vi "上管柱上转向轴合成.vi"() -> ()   [LabVIEW 2018]
uses:
  Global_Variable/Global.vi
  Database/Global1.vi
  Global_Variable/A131258.vi
  <vilib>/addons/database/Connection.llb/DB Tools Open Connec (String).vi
  <vilib>/addons/database/Connection.llb/Conn Execute.vi
  <vilib>/addons/database/Recordset.llb/Rec Fetch Recordset Data (R).vi
  <vilib>/Utility/config.llb/NI_LVConfig.lvlib
  <vilib>/addons/database/NI_Database_API.lvlib
panel:
  out "Fdeviceid":string
  out "USER_ID":string
  out "deviceid":string
  out "productid":string
  out "产品型号":string
  out "codeid":string
  out "联机模式":string
  out "用户权限":string
  out "用户名":string
  in  "上转向轴拉装报表":string[][](table)=[["mm"], ["mm/s"]]
  in  "上转向轴拉装判定结果":bool[][](array[boolean])=[[TRUE]]
  in  "选项卡控件 2":enum32{"上转向轴拉装曲线", "参数查看"}(tab)
  out "上序状态显示":string
  out "上序状态":bool
  in  "质量报警":bool
  in  "设备缺料":bool
  in  "设备故障":bool
  out "CCD卡簧检测":string
  out "判定结果3":string
  out "判定结果2":string
  out "判定结果1":string
  out "最终位移上限":dbl
  out "最终位移下限":dbl
  out "最小压力上限":dbl
  out "最小压力下限":dbl
  out "最大压力上限":dbl
  out "最大压力下限":dbl
  out "拉装最终位移(mm)":dbl
  out "不合格指示灯":bool
  out "合格指示灯":bool
  out "拉力位移曲线":cluster{dbl[], dbl[]}[](graph)
  out "位移区间内最大压力(KN)":dbl
  out "位移区间内最小压力(KN)":dbl
  out "产品条码":string
  in  "删除":bool
  in  "确定":bool
  in  "添加":bool
  in  "退出":bool
  in  "更新":bool
  in  "产品型号":string(combo)
  in  "选项卡控件 3":enum32{"上转向轴拉装参数", "产品管理", "用户管理"}(tab)
  in  "坐标轴参数":string[][](table)=[["mm"], ["mm/s"]]
  in  "判定框参数":string[][](table)=[["mm"], ["mm/s"]]
  in  "结果判定参数":string[][](table)=[["mm"], ["mm/s"]]
  in  "请输入添加的产品名称":string
  in  "请选择要删除的产品":string(combo)
  in  "进入用户管理":bool
  # "160上管柱上转向轴合成"
  # "下限值"
  # "上限值"
  # "拉装结果"
  # "判定结果"
  # "生产结果"
  # "产品二维码"
  # "上序状态："
  # "CCD卡簧检测结果"
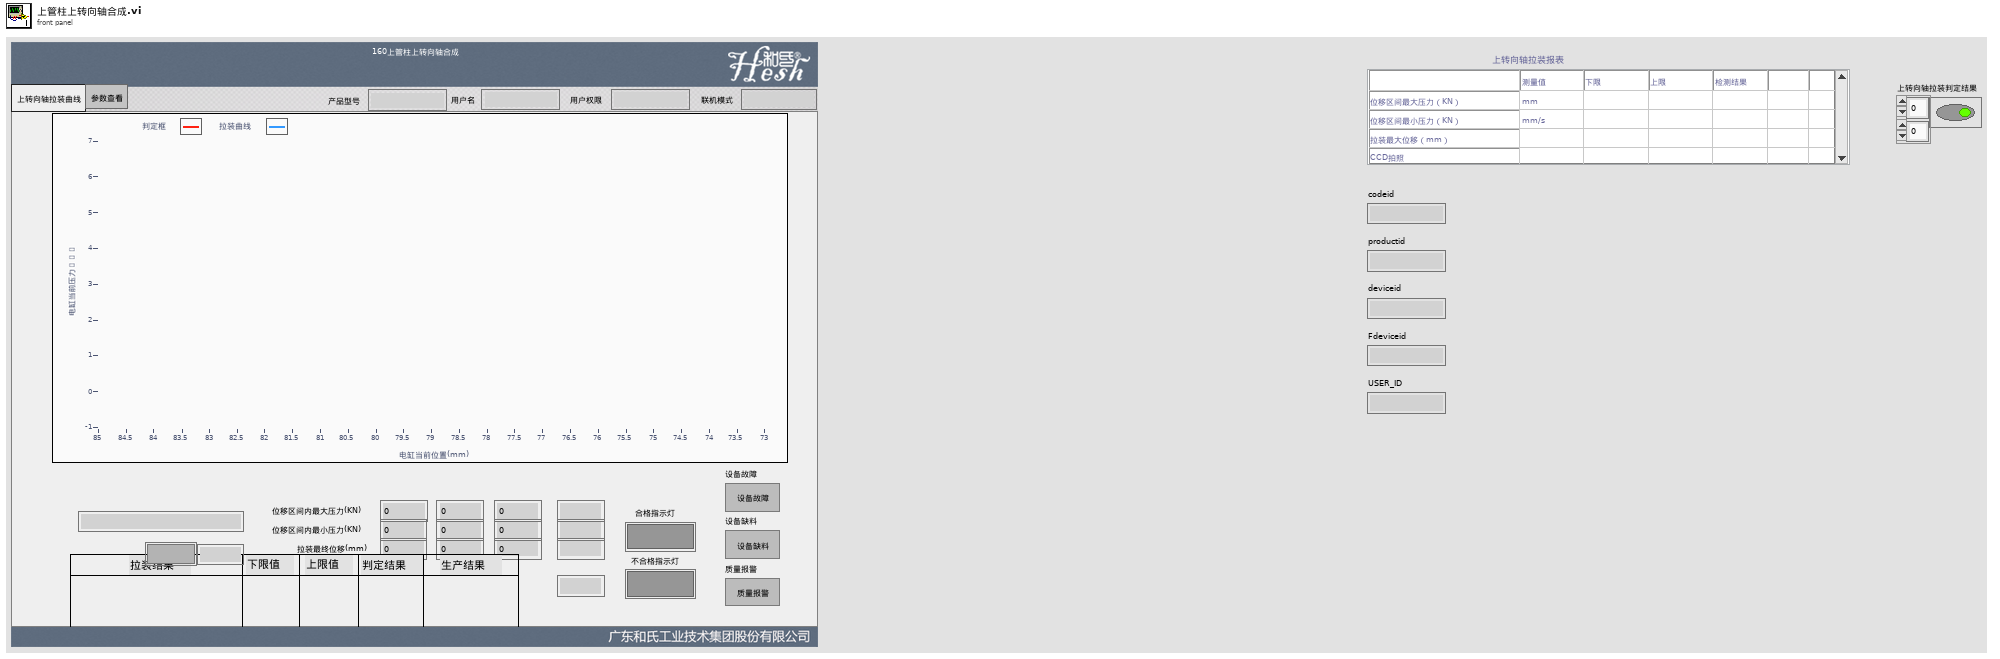
[diagram p1: front panel]
types:
  T1 = enum32{"Invalid", "Standard", "Closed", "Hidden", "Minimized", "Maximized"}
  T2 = cluster{"用户编号":string, "用户名":string, "用户密码(密文)":string, "用户权限":string}
  T3 = cluster{"设备名称":string, "用户名":string, "设备状态":enum16{"设备离线", "设备正常", "设备缺料", "设备故障", "质量报警"}, "附加信息":string}
  T4 = typedef "NI_LVConfig.lvlib/Config Data RefNum.ctl" = refnum<k1>
  T5 = cluster{i64, i64, string, "位移区间内最小压力(KN)":dbl, "最小压力下限":dbl, "最小压力上限":dbl, string, "判定结果2":string}
  T6 = cluster{i64, i64, string, "拉装最终位移(mm)":dbl, "最终位移下限":dbl, "最终位移上限":dbl, string, "判定结果3":string}
  T7 = cluster{i64, i64, string, dbl, dbl, dbl, string, "元素":string}
  T8 = cluster{i64, i64, string, "位移区间内最大压力(KN)":dbl, "最大压力下限":dbl, "最大压力上限":dbl, string, "判定结果1":string}
  T9 = cluster{i64, i64, string, "拉装最终位移(mm)":dbl, "最终位移下限":dbl, "最终位移上限":dbl, string, "元素":string}[]
  T10 = typedef "NI_Database_API.lvlib/Conn ObjectReference.ctl" = refnum<k1>
  T11 = cluster{i64, i64, "拉装最终位移(mm)":dbl, "最终位移下限":dbl, "最终位移上限":dbl, string, "元素":string}
  T12 = cluster{i64, i64, i64, string, "result string":string}
  T13 = cluster{i64, i64, i64, string, "result string":string}[]
  T14 = typedef "NI_Database_API.lvlib/Rec ObjectReference.ctl" = refnum<k1>
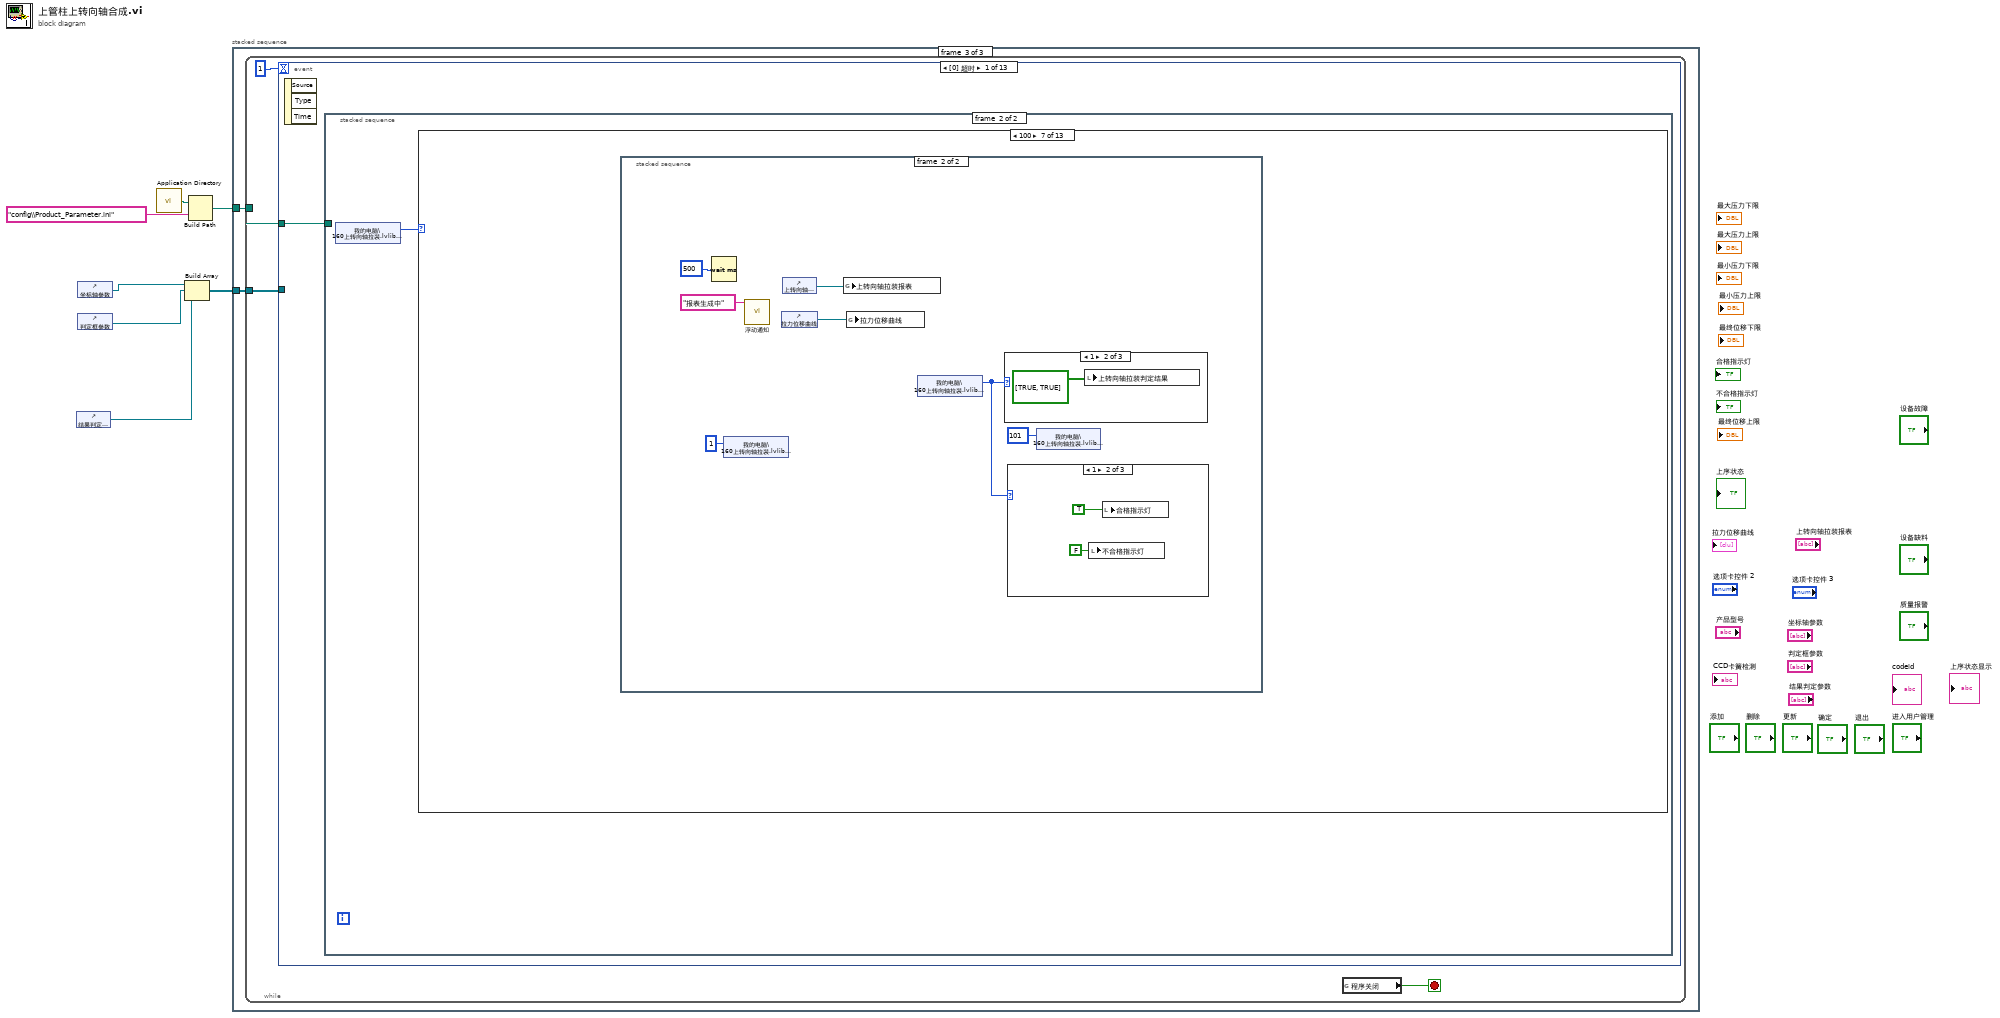
[diagram p0: block diagram]
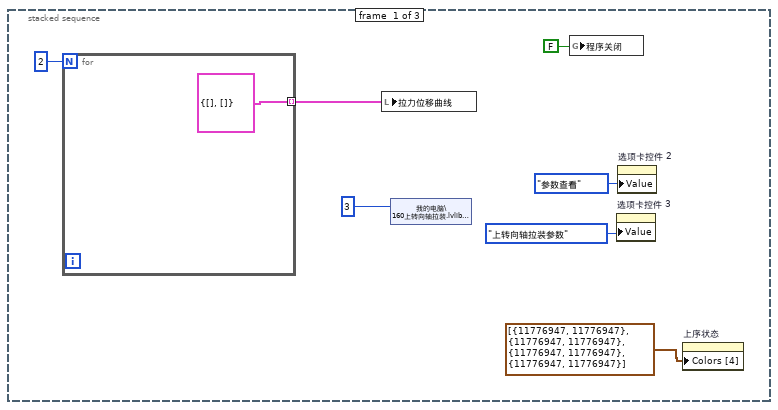
[diagram p2: hidden frame]
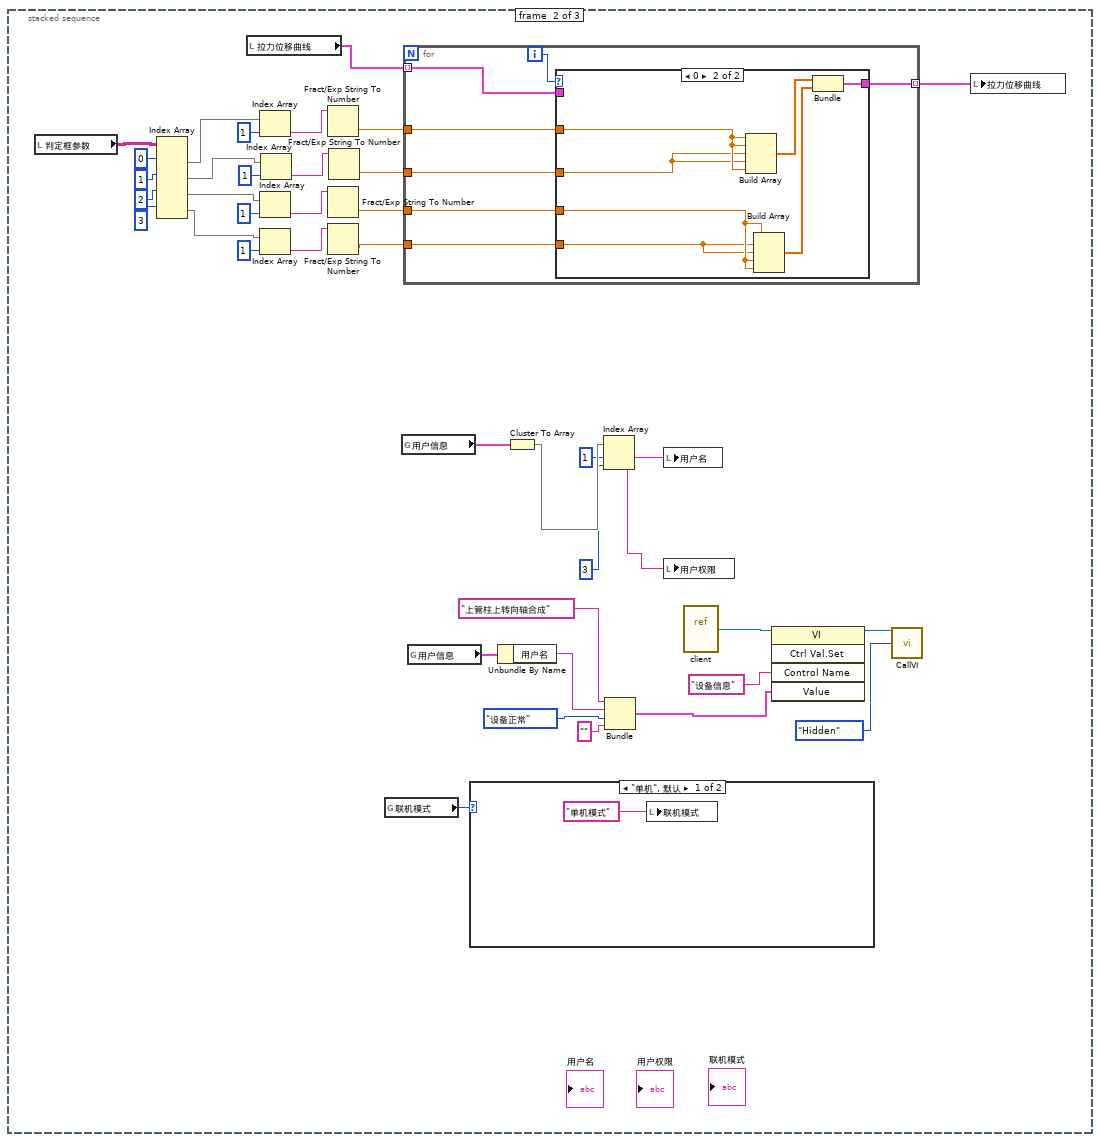
[diagram p3: hidden frame]
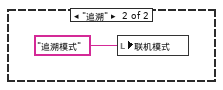
[diagram p4: hidden frame]
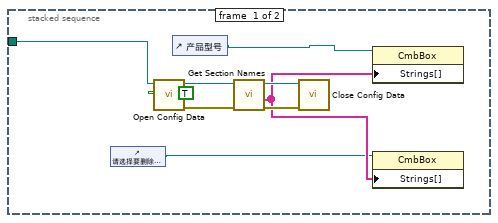
[diagram p6: hidden frame]
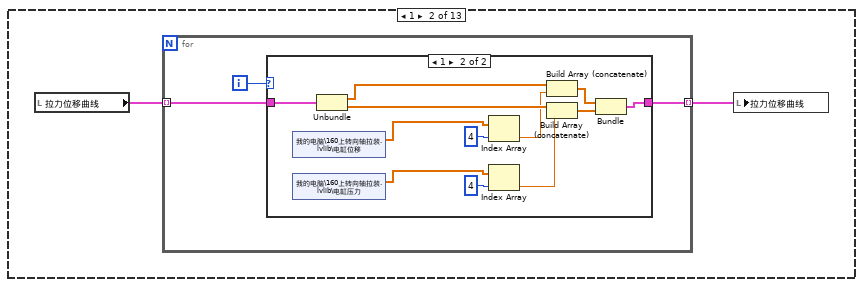
[diagram p8: hidden frame]
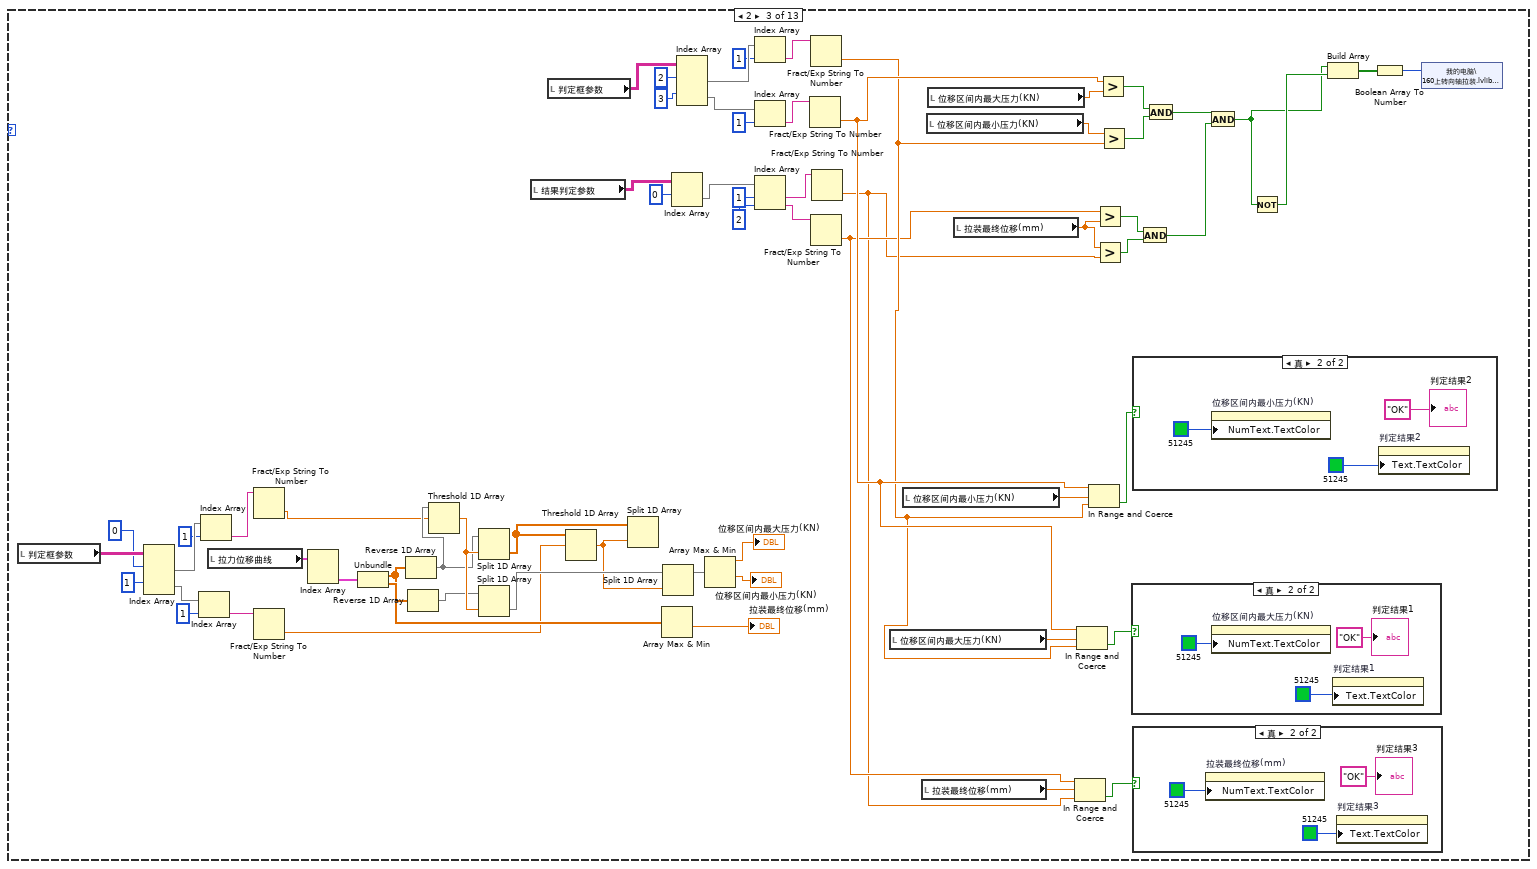
[diagram p10: hidden frame]
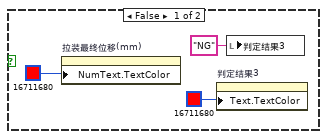
[diagram p11: hidden frame]
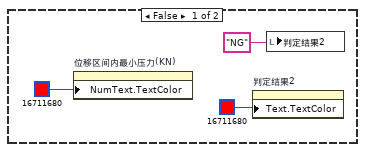
[diagram p12: hidden frame]
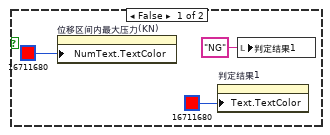
[diagram p13: hidden frame]
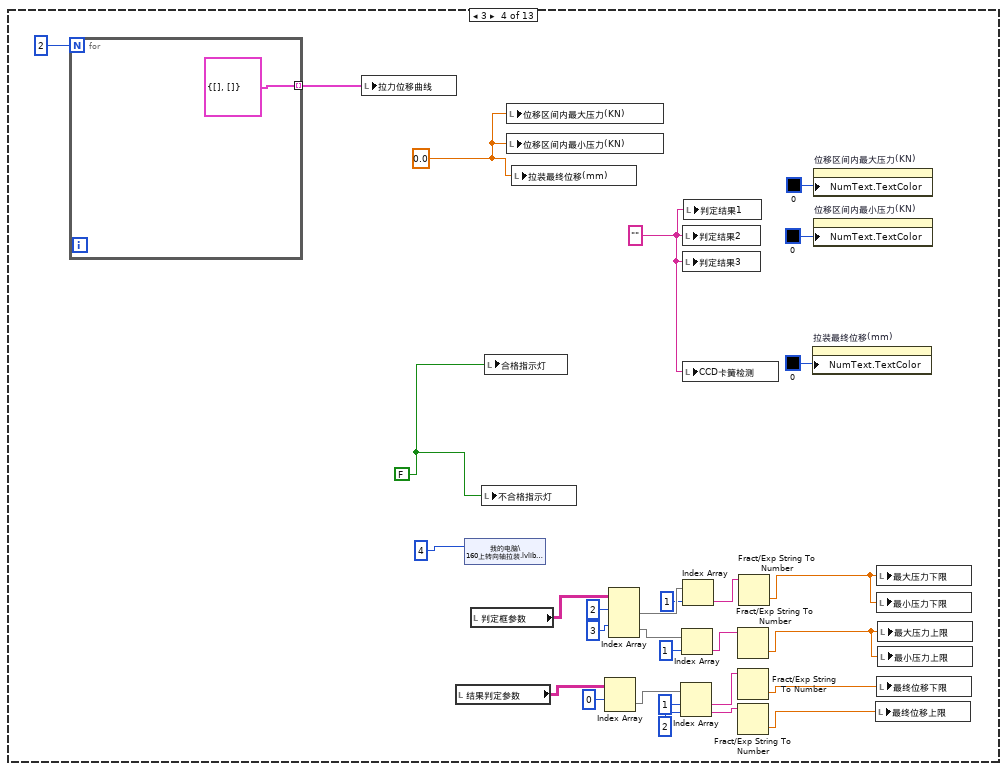
[diagram p14: hidden frame]
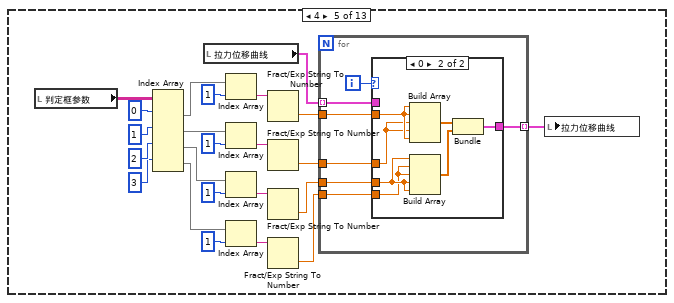
[diagram p15: hidden frame]
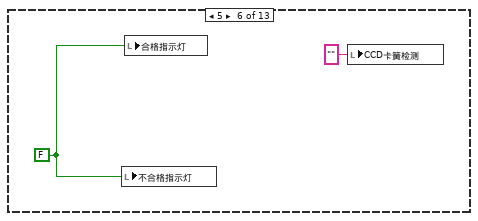
[diagram p17: hidden frame]
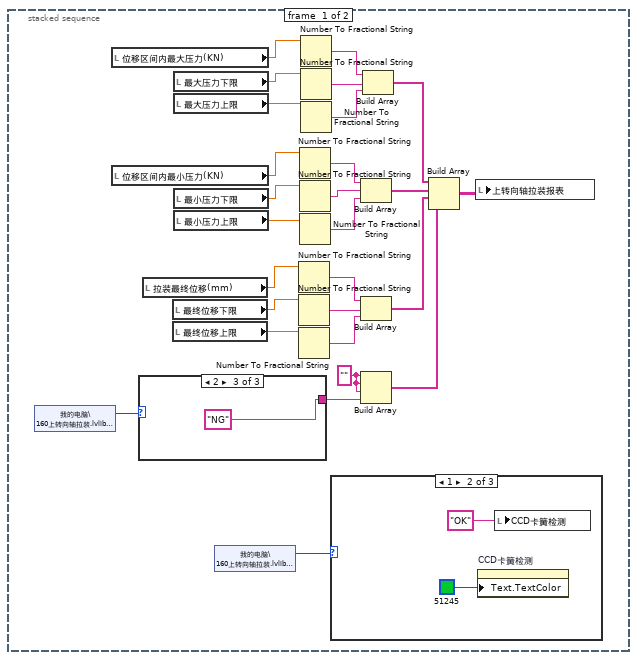
[diagram p18: hidden frame]
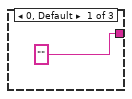
[diagram p19: hidden frame]
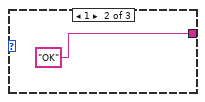
[diagram p20: hidden frame]
diagram:
  n1 = control-ref of="结果判定参数"() -> (w2:refnum<vi>)
  n2 = control-ref of="坐标轴参数"() -> (w4:refnum<vi>)
  n3 = control-ref of="判定框参数"() -> (w3:refnum<vi>)
  n4 = call <vilib>:"Application Directory.vi"() -> ("Application Directory"=w7:path)
  n5 = Build Array(w4, w3, w2) -> (w1:refnum<vi>[])
  n6 = Build Path(base path=w7, name or relative path="config\\Product_Parameter.ini" ("名称或相对路径")) -> (appended path=w5:path)
  n7 = stacked-sequence {
    tunnel: w5 -> [_ _ w74]
    tunnel: w1 -> [_ _ w73]
    frame #0 {
      n8 = for {
        N: 2 -> [_]
        tunnel: [cluster{dbl[], dbl[]} {[], []}] -> w14 mode=indexing
      }
      n9 = local write "拉力位移曲线"(w14) -> ()
      n10 = shared-variable "我的电脑\\160上转向轴拉装.lvlib\\备用_1"(3) -> ()  [unwired: 1 in, 1 out]
      n11 = global write "Global.vi" "程序关闭"(FALSE ("程序关闭")) -> ()
      n12 = property on="选项卡控件 3" class="TabCtl (严格)"("Value"=enum32{"上转向轴拉装参数", "产品管理", "用户管理"}."上转向轴拉装参数" ("选项卡控件 3")) -> ()  [unwired: 2 in, 2 out]
      n13 = property on="选项卡控件 2" class="TabCtl (严格)"("Value"=enum32{"上转向轴拉装曲线", "参数查看"}."参数查看" ("选项卡控件 2")) -> ()  [unwired: 2 in, 2 out]
      n14 = property on="上序状态" class="Bool (严格)"("Colors [4]"=cluster{u32, u32}[] [{11776947, 11776947}, {11776947, 11776947}, {11776947, 11776947}, {11776947, 11776947}] ("颜色[4]")) -> ()  [unwired: 2 in, 2 out]
    }
    frame #1 {
      n15 = local read "判定框参数"() -> (w53:string[][])
      n16 = Index Array(array=w53, index (row) #1=0 ("索引 (行)"), index (row) #2=1 ("索引 (行)"), index (row) #3=2 ("索引 (行)"), index (row) #4=3 ("索引 (行)")) -> (element #1=w48:string[], element #2=w43:string[], element #3=w38:string[], element #4=w34:string[])  [unwired: 4 in]
      n17 = local read "拉力位移曲线"() -> (w55:cluster{dbl[], dbl[]}[])
      n18 = Index Array(array=w48, index=1 ("索引")) -> (element=w46:string)
      n19 = Index Array(array=w38, index=1 ("索引")) -> (element=w39:string)
      n20 = Index Array(array=w34, index=1 ("索引")) -> (element=w35:string)
      n21 = Index Array(array=w43, index=1 ("索引")) -> (element=w42:string)
      n22 = Fract/Exp String To Number(string=w46) -> (number=w45:dbl)  [unwired: 3 in, 1 out]
      n23 = Fract/Exp String To Number(string=w39) -> (number=w37:dbl)  [unwired: 3 in, 1 out]
      n24 = Fract/Exp String To Number(string=w35) -> (number=w33:dbl)  [unwired: 3 in, 1 out]
      n25 = Fract/Exp String To Number(string=w42) -> (number=w41:dbl)  [unwired: 3 in, 1 out]
      n26 = global read "Global1.vi" "联机模式"() -> (w27:enum16{"单机", "追溯"})
      n27 = global read "Global1.vi" "用户信息"() -> (w23:T2)
      n28 = for {
        tunnel: [w64] -> w54 mode=indexing
        tunnel: w55 -> [w63] mode=indexing
        tunnel: w45 -> [w61]
        tunnel: w41 -> [w60]
        tunnel: w37 -> [w59]
        tunnel: w33 -> [w58]
        i -> [w62]
        n29 = case shown="0" w62 {
          tunnel: [w65 w70] -> w64
          tunnel: w63 -> [w65 _]
          tunnel: w61 -> [_ w69]
          tunnel: w60 -> [_ w68]
          tunnel: w59 -> [_ w67]
          tunnel: w58 -> [_ w66]
          frame Default {
          }
          frame 0 {
            n30 = Build Array(w69, w69, w68, w68, w69) -> (w71:dbl[])
            n31 = Build Array(w67, w66, w66, w67, w67) -> (w72:dbl[])
            n32 = Bundle(w71, w72) -> (w70:cluster{dbl[], dbl[]})  [unwired: 1 in]
          }
        }
      }
      n33 = global read "Global1.vi" "用户信息"() -> (w30:T2)
      n34 = case shown="\"单机\", 默认" w27 {
        frame "单机", Default {
          n35 = local write "联机模式"("单机模式" ("联机模式")) -> ()
        }
        frame "追溯" {
          n36 = local write "联机模式"("追溯模式" ("联机模式")) -> ()
        }
      }
      n37 = Unbundle By Name(w30) -> ("用户名"=w31:string)
      n38 = Cluster To Array(cluster=w23) -> (array=w24:string[])
      n39 = Index Array(array=w24, index #1=1 ("索引"), index #2=3 ("索引")) -> (element #1=w25:string, element #2=w26:string)
      n40 = Bundle("设备名称"="上管柱上转向轴合成", "用户名"=w31, "设备状态"=enum16{"设备离线", "设备正常", "设备缺料", "设备故障", "质量报警"}."设备正常", "附加信息"="") -> (w32:T3)  [unwired: 1 in]
      n41 = local write "用户名"(w25) -> ()
      n42 = local write "用户权限"(w26) -> ()
      n43 = vi-ref "client.vi"() -> (w28:refnum<vi>)
      n44 = invoke class="VI" method="Ctrl Val.Set"(reference=w28, "Control Name"="设备信息" ("控件名"), "Value"=w32) -> (reference out=w29:refnum<vi>)  [unwired: 2 in, 4 out]
      n45 = call "CallVI.vi"("VI引用"=w29, "状态"=T1."Hidden") -> ()  [unwired: 11 in, 3 out]
      n46 = local write "拉力位移曲线"(w54) -> ()
    }
    frame #2 {
      n47 = while {
        tunnel: w74 -> [w77]
        tunnel: w73 -> [w78]
        stop <- w75 stop-if-true
        n48 = event shown="[0] 超时" {
          selector: _ -> [_ _ _ _ _ _ _ _ _ _ _ _ _]
          dyn-events: _ -> [_ _ _ _ _ _ _ _ _ _ _ _ _]
          timeout: 1 -> [_ _ _ _ _ _ _ _ _ _ _ _ _]
          tunnel: w77 -> [w79 w546 _ w679 w696 _ w707 _ _ _ _ _ _]
          tunnel: w78 -> [_ _ _ w677 w695 _ w706 _ _ _ _ _ _]
          event Timeout {
            n49 = event-data() -> ()  [unwired: 1 in, 3 out]
            n50 = stacked-sequence {
              tunnel: w79 -> [w82 _]
              frame #0 {
                n51 = control-ref of="请选择要删除的产品"() -> (w81:refnum<vi>)
                n52 = call <vilib>:"Open Config Data.vi"("create file if necessary (T)"=TRUE, "configuration file path"=w82) -> ("error out"=w85:errorcluster, "refnum"=w84:T4)  [unwired: 7 in, 1 out]
                n53 = control-ref of="产品型号"() -> (w80:refnum<vi>)
                n54 = call <vilib>:"Get Section Names.vi"("error in (no error)"=w85, "refnum"=w84) -> ("error out"=w87:errorcluster, "section names"=w83:string[], "refnum out"=w86:T4)  [unwired: 7 in]
                n55 = call <vilib>:"Close Config Data.vi"("error in (no error)"=w87, "refnum"=w86) -> ()  [unwired: 8 in, 2 out]
                n56 = property on="属性节点" class="CmbBox"(reference=w80, "Strings[]"=w83) -> ()  [unwired: 1 in, 2 out]
                n57 = property on="属性节点" class="CmbBox"(reference=w81, "Strings[]"=w83) -> ()  [unwired: 1 in, 2 out]
              }
              frame #1 {
                n58 = shared-variable "我的电脑\\160上转向轴拉装.lvlib\\备用_1"() -> (w89:u16)  [unwired: 1 in, 1 out]
                n59 = case shown="100" w89 {
                  frame 0, Default {
                  }
                  frame 1 {
                    n60 = local read "拉力位移曲线"() -> (w90:cluster{dbl[], dbl[]}[])
                    n61 = for {
                      tunnel: [w94] -> w91 mode=indexing
                      tunnel: w90 -> [w93] mode=indexing
                      i -> [w92]
                      n62 = case shown="1" w92 {
                        tunnel: [w95 w101] -> w94
                        tunnel: w93 -> [w95 w100]
                        frame Default {
                        }
                        frame 1 {
                          n63 = shared-variable "我的电脑\\160上转向轴拉装.lvlib\\电缸位移"() -> (w96:sgl[])  [unwired: 1 in, 1 out]
                          n64 = shared-variable "我的电脑\\160上转向轴拉装.lvlib\\电缸压力"() -> (w97:sgl[])  [unwired: 1 in, 1 out]
                          n65 = Unbundle(w100) -> (w105:dbl[], w104:dbl[])
                          n66 = Index Array(array=w96, index=4) -> (element=w98:sgl)
                          n67 = Index Array(array=w97, index=4) -> (element=w99:sgl)
                          n68 = Build Array (concatenate)(w105, w98) -> (w103:dbl[])
                          n69 = Build Array (concatenate)(w104, w99) -> (w102:dbl[])
                          n70 = Bundle(w103, w102) -> (w101:cluster{dbl[], dbl[]})  [unwired: 1 in]
                        }
                      }
                    }
                    n71 = local write "拉力位移曲线"(w91) -> ()
                  }
                  frame 2 {
                    n72 = local read "判定框参数"() -> (w138:string[][])
                    n73 = Index Array(array=w138, index (row) #1=0 ("索引 (行)"), index (row) #2=1 ("索引 (行)")) -> (element #1=w135:string[], element #2=w133:string[])  [unwired: 2 in]
                    n74 = Index Array(array=w133, index=1 ("索引")) -> (element=w129:string)
                    n75 = Index Array(array=w135, index=1 ("索引")) -> (element=w131:string)
                    n76 = local read "拉力位移曲线"() -> (w171:cluster{dbl[], dbl[]}[])
                    n77 = Fract/Exp String To Number(string=w131) -> (number=w130:dbl)  [unwired: 3 in, 1 out]
                    n78 = Fract/Exp String To Number(string=w129) -> (number=w128:dbl)  [unwired: 3 in, 1 out]
                    n79 = Index Array(array=w171) -> (element #2=w157:cluster{dbl[], dbl[]})  [unwired: 2 in, 1 out]
                    n80 = Unbundle(w157) -> (w152:dbl[], w161:dbl[])
                    n81 = Reverse 1D Array(array=w152) -> (reversed array=w162:dbl[])
                    n82 = Reverse 1D Array(array=w161) -> (reversed array=w160:dbl[])
                    n83 = Threshold 1D Array(2:w130, 3:w162) -> (0:w170:dbl)  [unwired: 1 in]
                    n84 = Split 1D Array(array=w162, index=w170) -> (second subarray=w168:dbl[])  [unwired: 1 out]
                    n85 = Split 1D Array(array=w160, index=w170) -> (second subarray=w169:dbl[])  [unwired: 1 out]
                    n86 = local read "结果判定参数"() -> (w118:string[][])
                    n87 = local read "判定框参数"() -> (w126:string[][])
                    n88 = Threshold 1D Array(2:w128, 3:w168) -> (0:w167:dbl)  [unwired: 1 in]
                    n89 = Split 1D Array(array=w168, index=w167) -> ()  [unwired: 2 out]
                    n90 = Array Max & Min(array=w152) -> (min value=→"拉装最终位移(mm)":dbl)  [unwired: 3 out]
                    n91 = Split 1D Array(array=w169, index=w167) -> (first subarray=w163:dbl[])  [unwired: 1 out]
                    n92 = Index Array(array=w118, index (row)=0 ("索引 (行)")) -> (element=w116:string[])  [unwired: 1 in]
                    n93 = Index Array(array=w126, index (row) #1=2 ("索引 (行)"), index (row) #2=3 ("索引 (行)")) -> (element #1=w124:string[], element #2=w122:string[])  [unwired: 2 in]
                    n94 = Array Max & Min(array=w163) -> (max value=→"位移区间内最大压力(KN)":dbl, min value=→"位移区间内最小压力(KN)":dbl)  [unwired: 2 out]
                    n95 = Index Array(array=w124, index=1 ("索引")) -> (element=w119:string)
                    n96 = Index Array(array=w122, index=1 ("索引")) -> (element=w120:string)
                    n97 = Index Array(array=w116, index #1=1 ("索引"), index #2=2 ("索引")) -> (element #1=w113:string, element #2=w112:string)
                    n98 = Fract/Exp String To Number(string=w120) -> (number=w111:dbl)  [unwired: 3 in, 1 out]
                    n99 = Fract/Exp String To Number(string=w119) -> (number=w110:dbl)  [unwired: 3 in, 1 out]
                    n100 = Fract/Exp String To Number(string=w112) -> (number=w109:dbl)  [unwired: 3 in, 1 out]
                    n101 = Fract/Exp String To Number(string=w113) -> (number=w108:dbl)  [unwired: 3 in, 1 out]
                    n102 = local read "位移区间内最大压力(KN)"() -> (w144:dbl)
                    n103 = local read "位移区间内最小压力(KN)"() -> (w142:dbl)
                    n104 = local read "拉装最终位移(mm)"() -> (w140:dbl)
                    n105 = local read "位移区间内最小压力(KN)"() -> (w155:dbl)
                    n106 = local read "位移区间内最大压力(KN)"() -> (w156:dbl)
                    n107 = local read "拉装最终位移(mm)"() -> (w150:dbl)
                    n108 = In Range and Coerce(upper limit=w109, x=w140, lower limit=w108) -> (In Range?=w139:bool)  [unwired: 1 out]
                    n109 = In Range and Coerce(upper limit=w111, x=w144, lower limit=w110) -> (In Range?=w143:bool)  [unwired: 1 out]
                    n110 = In Range and Coerce(upper limit=w111, x=w142, lower limit=w110) -> (In Range?=w141:bool)  [unwired: 1 out]
                    n111 = Greater?(x=w109, y=w150) -> (0:w149:bool)
                    n112 = Greater?(x=w150, y=w108) -> (0:w148:bool)
                    n113 = Greater?(x=w111, y=w156) -> (0:w154:bool)
                    n114 = Greater?(x=w155, y=w110) -> (0:w153:bool)
                    n115 = case shown="真" w143 {
                      frame False {
                        n116 = property on="位移区间内最大压力(KN)" class="DigNum (严格)"("NumText.TextColor"=u32 16711680) -> ()  [unwired: 2 in, 2 out]
                        n117 = property on="判定结果1" class="Str"("Text.TextColor"=u32 16711680) -> ()  [unwired: 2 in, 2 out]
                        n118 = local write "判定结果1"("NG" ("判定结果1")) -> ()
                      }
                      frame True {
                        n119 = property on="位移区间内最大压力(KN)" class="DigNum (严格)"("NumText.TextColor"=u32 51245) -> ()  [unwired: 2 in, 2 out]
                        n120 = property on="判定结果1" class="Str"("Text.TextColor"=u32 51245) -> ()  [unwired: 2 in, 2 out]
                        "判定结果1" <- "OK" ("判定结果1")
                      }
                    }
                    n121 = case shown="真" w141 {
                      frame False {
                        n122 = property on="位移区间内最小压力(KN)" class="DigNum (严格)"("NumText.TextColor"=u32 16711680) -> ()  [unwired: 2 in, 2 out]
                        n123 = property on="判定结果2" class="Str"("Text.TextColor"=u32 16711680) -> ()  [unwired: 2 in, 2 out]
                        n124 = local write "判定结果2"("NG" ("判定结果1")) -> ()
                      }
                      frame True {
                        n125 = property on="位移区间内最小压力(KN)" class="DigNum (严格)"("NumText.TextColor"=u32 51245) -> ()  [unwired: 2 in, 2 out]
                        n126 = property on="判定结果2" class="Str"("Text.TextColor"=u32 51245) -> ()  [unwired: 2 in, 2 out]
                        "判定结果2" <- "OK" ("判定结果1")
                      }
                    }
                    n127 = case shown="真" w139 {
                      frame False {
                        n128 = property on="拉装最终位移(mm)" class="DigNum (严格)"("NumText.TextColor"=u32 16711680) -> ()  [unwired: 2 in, 2 out]
                        n129 = property on="判定结果3" class="Str"("Text.TextColor"=u32 16711680) -> ()  [unwired: 2 in, 2 out]
                        n130 = local write "判定结果3"("NG" ("判定结果3")) -> ()
                      }
                      frame True {
                        n131 = property on="拉装最终位移(mm)" class="DigNum (严格)"("NumText.TextColor"=u32 51245) -> ()  [unwired: 2 in, 2 out]
                        n132 = property on="判定结果3" class="Str"("Text.TextColor"=u32 51245) -> ()  [unwired: 2 in, 2 out]
                        "判定结果3" <- "OK" ("判定结果3")
                      }
                    }
                    n133 = And(x=w149, y=w148) -> (x .and. y?=w146:bool)
                    n134 = And(x=w154, y=w153) -> (x .and. y?=w147:bool)
                    n135 = And(x=w147, y=w146) -> (x .and. y?=w145:bool)
                    n136 = Not(x=w145) -> (.not. x?=w164:bool)
                    n137 = Build Array(w145, w164) -> (w166:bool[])
                    n138 = Boolean Array To Number(Boolean array=w166) -> (number=w165:u32)
                    n139 = shared-variable "我的电脑\\160上转向轴拉装.lvlib\\备用_2"(w165) -> ()  [unwired: 1 in, 1 out]
                  }
                  frame 3 {
                    w190 = "" ("判定结果2")
                    w215 = FALSE
                    w211 = 0.0
                    n140 = for {
                      N: 2 -> [_]
                      tunnel: [cluster{dbl[], dbl[]} {[], []}] -> w218 mode=indexing
                    }
                    n141 = local write "拉力位移曲线"(w218) -> ()
                    n142 = local read "结果判定参数"() -> (w199:string[][])
                    n143 = shared-variable "我的电脑\\160上转向轴拉装.lvlib\\备用_1"(4) -> ()  [unwired: 1 in, 1 out]
                    n144 = local read "判定框参数"() -> (w210:string[][])
                    n145 = local write "不合格指示灯"(w215) -> ()
                    n146 = local write "合格指示灯"(w215) -> ()
                    n147 = local write "位移区间内最大压力(KN)"(w211) -> ()
                    n148 = local write "位移区间内最小压力(KN)"(w211) -> ()
                    n149 = local write "拉装最终位移(mm)"(w211) -> ()
                    n150 = Index Array(array=w199, index (row)=0 ("索引 (行)")) -> (element=w197:string[])  [unwired: 1 in]
                    n151 = Index Array(array=w210, index (row) #1=2 ("索引 (行)"), index (row) #2=3 ("索引 (行)")) -> (element #1=w207:string[], element #2=w205:string[])  [unwired: 2 in]
                    n152 = Index Array(array=w197, index #1=1 ("索引"), index #2=2 ("索引")) -> (element #1=w194:string, element #2=w193:string)
                    n153 = Index Array(array=w205, index=1 ("索引")) -> (element=w202:string)
                    n154 = local write "判定结果2"(w190) -> ()
                    n155 = local write "判定结果3"(w190) -> ()
                    n156 = local write "CCD卡簧检测"(w190) -> ()
                    n157 = Index Array(array=w207, index=1 ("索引")) -> (element=w203:string)
                    n158 = local write "判定结果1"(w190) -> ()
                    n159 = Fract/Exp String To Number(string=w202) -> (number=w200:dbl)  [unwired: 3 in, 1 out]
                    n160 = Fract/Exp String To Number(string=w194) -> (number=w192:dbl)  [unwired: 3 in, 1 out]
                    n161 = Fract/Exp String To Number(string=w193) -> (number=w191:dbl)  [unwired: 3 in, 1 out]
                    n162 = Fract/Exp String To Number(string=w203) -> (number=w201:dbl)  [unwired: 3 in, 1 out]
                    n163 = property on="拉装最终位移(mm)" class="DigNum (严格)"("NumText.TextColor"=u32 0) -> ()  [unwired: 2 in, 2 out]
                    n164 = property on="位移区间内最大压力(KN)" class="DigNum (严格)"("NumText.TextColor"=u32 0) -> ()  [unwired: 2 in, 2 out]
                    n165 = property on="位移区间内最小压力(KN)" class="DigNum (严格)"("NumText.TextColor"=u32 0) -> ()  [unwired: 2 in, 2 out]
                    n166 = local write "最终位移上限"(w191) -> ()
                    n167 = local write "最大压力下限"(w201) -> ()
                    n168 = local write "最小压力下限"(w201) -> ()
                    n169 = local write "最终位移下限"(w192) -> ()
                    n170 = local write "最大压力上限"(w200) -> ()
                    n171 = local write "最小压力上限"(w200) -> ()
                  }
                  frame 4 {
                    n172 = local read "判定框参数"() -> (w224:string[][])
                    n173 = Index Array(array=w224, index (row) #1=0 ("索引 (行)"), index (row) #2=1 ("索引 (行)"), index (row) #3=2 ("索引 (行)"), index (row) #4=3 ("索引 (行)")) -> (element #1=w236:string[], element #2=w232:string[], element #3=w228:string[], element #4=w225:string[])  [unwired: 4 in]
                    n174 = local read "拉力位移曲线"() -> (w241:cluster{dbl[], dbl[]}[])
                    n175 = Index Array(array=w236, index=1 ("索引")) -> (element=w234:string)
                    n176 = Index Array(array=w232, index=1 ("索引")) -> (element=w231:string)
                    n177 = Index Array(array=w228, index=1 ("索引")) -> (element=w229:string)
                    n178 = Index Array(array=w225, index=1 ("索引")) -> (element=w226:string)
                    n179 = Fract/Exp String To Number(string=w234) -> (number=w223:dbl)  [unwired: 3 in, 1 out]
                    n180 = Fract/Exp String To Number(string=w231) -> (number=w222:dbl)  [unwired: 3 in, 1 out]
                    n181 = Fract/Exp String To Number(string=w229) -> (number=w221:dbl)  [unwired: 3 in, 1 out]
                    n182 = Fract/Exp String To Number(string=w226) -> (number=w220:dbl)  [unwired: 3 in, 1 out]
                    n183 = for {
                      tunnel: [w249] -> w242 mode=indexing
                      tunnel: w241 -> [w248] mode=indexing
                      tunnel: w223 -> [w246]
                      tunnel: w222 -> [w245]
                      tunnel: w221 -> [w244]
                      tunnel: w220 -> [w243]
                      i -> [w247]
                      n184 = case shown="0" w247 {
                        tunnel: [w250 w255] -> w249
                        tunnel: w248 -> [w250 _]
                        tunnel: w246 -> [_ w254]
                        tunnel: w245 -> [_ w253]
                        tunnel: w244 -> [_ w252]
                        tunnel: w243 -> [_ w251]
                        frame Default {
                        }
                        frame 0 {
                          n185 = Build Array(w254, w254, w253, w253, w254) -> (w256:dbl[])
                          n186 = Build Array(w252, w251, w251, w252, w252) -> (w257:dbl[])
                          n187 = Bundle(w256, w257) -> (w255:cluster{dbl[], dbl[]})  [unwired: 1 in]
                        }
                      }
                    }
                    n188 = local write "拉力位移曲线"(w242) -> ()
                  }
                  frame 5 {
                    w259 = FALSE
                    n189 = local write "不合格指示灯"(w259) -> ()
                    n190 = local write "合格指示灯"(w259) -> ()
                    n191 = local write "CCD卡簧检测"("" ("CCD卡簧检测")) -> ()
                  }
                  frame 100 {
                    n192 = stacked-sequence {
                      frame #0 {
                        w260 = "" ("元素")
                        n193 = shared-variable "我的电脑\\160上转向轴拉装.lvlib\\备用_4"() -> (w283:u16)  [unwired: 1 in, 1 out]
                        n194 = local read "位移区间内最大压力(KN)"() -> (w274:dbl)
                        n195 = local read "位移区间内最小压力(KN)"() -> (w279:dbl)
                        n196 = case shown="2" w283 {
                          tunnel: ["" ("元素") "OK" "NG"] -> w285
                          frame 0, Default {
                          }
                          frame 1 {
                          }
                          frame 2 {
                          }
                        }
                        n197 = local read "拉装最终位移(mm)"() -> (w282:dbl)
                        n198 = local read "最终位移下限"() -> (w281:dbl)
                        n199 = local read "最终位移上限"() -> (w280:dbl)
                        n200 = local read "最大压力下限"() -> (w275:dbl)
                        n201 = local read "最大压力上限"() -> (w276:dbl)
                        n202 = local read "最小压力下限"() -> (w278:dbl)
                        n203 = local read "最小压力上限"() -> (w277:dbl)
                        n204 = shared-variable "我的电脑\\160上转向轴拉装.lvlib\\备用_4"() -> (w286:u16)  [unwired: 1 in, 1 out]
                        n205 = Number To Fractional String(number=w282) -> (F-format string=w267:string)  [unwired: 3 in]
                        n206 = Number To Fractional String(number=w281) -> (F-format string=w268:string)  [unwired: 3 in]
                        n207 = Number To Fractional String(number=w280) -> (F-format string=w269:string)  [unwired: 3 in]
                        n208 = Number To Fractional String(number=w279) -> (F-format string=w264:string)  [unwired: 3 in]
                        n209 = Number To Fractional String(number=w278) -> (F-format string=w265:string)  [unwired: 3 in]
                        n210 = Number To Fractional String(number=w277) -> (F-format string=w266:string)  [unwired: 3 in]
                        n211 = Number To Fractional String(number=w274) -> (F-format string=w261:string)  [unwired: 3 in]
                        n212 = Number To Fractional String(number=w275) -> (F-format string=w262:string)  [unwired: 3 in]
                        n213 = Number To Fractional String(number=w276) -> (F-format string=w263:string)  [unwired: 3 in]
                        n214 = case shown="1" w286 {
                          frame 0, Default {
                          }
                          frame 1 {
                            n215 = property on="CCD卡簧检测" class="Str"("Text.TextColor"=u32 51245) -> ()  [unwired: 2 in, 2 out]
                            n216 = local write "CCD卡簧检测"("OK") -> ()
                          }
                          frame 2 {
                            n217 = property on="CCD卡簧检测" class="Str"("Text.TextColor"=u32 16711680) -> ()  [unwired: 2 in, 2 out]
                            n218 = local write "CCD卡簧检测"("NG") -> ()
                          }
                        }
                        n219 = Build Array(w264, w265, w266) -> (w270:string[])
                        n220 = Build Array(w267, w268, w269) -> (w272:string[])
                        n221 = Build Array(w260, w260, w260, w285) -> (w284:string[])
                        n222 = Build Array(w261, w262, w263) -> (w271:string[])
                        n223 = Build Array(w271, w270, w272, w284) -> (w273:string[][])
                        n224 = local write "上转向轴拉装报表"(w273) -> ()
                      }
                      frame #1 {
                        n225 = Wait (ms)(milliseconds to wait=u32 500 ("等待时间（毫秒）")) -> ()  [unwired: 1 out]
                        n226 = shared-variable "我的电脑\\160上转向轴拉装.lvlib\\备用_3"(u16 1 ("备用1")) -> ()  [unwired: 1 in, 1 out]
                        n227 = call "浮动通知.vi"("通知内容"="报表生成中" ("Status")) -> ()  [unwired: 11 in]
                        n228 = control-ref of="拉力位移曲线"() -> (w296:refnum<vi>)
                        n229 = control-ref of="上转向轴拉装报表"() -> (w297:refnum<vi>)
                        n230 = global write "Global.vi" "上转向轴拉装报表"(w297) -> ()
                        n231 = global write "A131258.vi" "拉力位移曲线"(w296) -> ()
                        n232 = shared-variable "我的电脑\\160上转向轴拉装.lvlib\\备用_5"() -> (w295:u16)  [unwired: 1 in, 1 out]
                        n233 = case shown="1" w295 {
                          frame 0, Default {
                          }
                          frame 1 {
                            n234 = local write "上转向轴拉装判定结果"(bool[][] [[TRUE, TRUE]] ("判定结果")) -> ()
                          }
                          frame 2 {
                            n235 = local write "上转向轴拉装判定结果"(bool[][] [[TRUE, FALSE]] ("判定结果")) -> ()
                          }
                        }
                        n236 = case shown="1" w295 {
                          frame 0, Default {
                          }
                          frame 1 {
                            n237 = local write "不合格指示灯"(FALSE ("不合格指示灯")) -> ()
                            n238 = local write "合格指示灯"(TRUE) -> ()
                          }
                          frame 2 {
                            n239 = local write "不合格指示灯"(TRUE) -> ()
                            n240 = local write "合格指示灯"(FALSE ("合格指示灯")) -> ()
                          }
                        }
                        n241 = shared-variable "我的电脑\\160上转向轴拉装.lvlib\\备用_1"(u16 101 ("备用1")) -> ()  [unwired: 1 in, 1 out]
                      }
                    }
                  }
                  frame 101 {
                    n242 = shared-variable "我的电脑\\Global.lvlib\\工位追溯码"() -> (w310:string)  [unwired: 1 in, 1 out]
                    n243 = shared-variable "我的电脑\\160上转向轴拉装.lvlib\\备用_1"(u16 102 ("备用1")) -> ()  [unwired: 1 in, 1 out]
                    n244 = Wait (ms)(milliseconds to wait=u32 800 ("等待时间（毫秒）")) -> ()  [unwired: 1 out]
                    n245 = call "Report_A131258.vi"("文件重命名"=TRUE, "文件名称"=w310, "布尔数组"="上转向轴拉装判定结果") -> ()  [unwired: 8 in, 1 out]
                  }
                  frame 102 {
                    n246 = global read "Global1.vi" "联机模式"() -> (w312:enum16{"单机", "追溯"})
                    n247 = case shown="\"追溯\"" w312 {
                      frame "单机", Default {
                        n248 = shared-variable "我的电脑\\160上转向轴拉装.lvlib\\备用_1"(u16 103 ("备用1")) -> ()  [unwired: 1 in, 1 out]
                      }
                      frame "追溯" {
                        n249 = stacked-sequence {
                          frame #0 {
                            w317 = 0.0
                            n250 = local read "位移区间内最小压力(KN)"() -> (w340:dbl)
                            n251 = local read "拉装最终位移(mm)"() -> (w348:dbl)
                            n252 = local read "deviceid"() -> (w336:string)
                            n253 = local read "codeid"() -> (w339:string)
                            n254 = local read "deviceid"() -> (w344:string)
                            n255 = local read "codeid"() -> (w347:string)
                            n256 = local read "最小压力上限"() -> (w342:dbl)
                            n257 = local read "最小压力下限"() -> (w341:dbl)
                            n258 = shared-variable "我的电脑\\160上转向轴拉装.lvlib\\备用_4"() -> (w316:u16)  [unwired: 1 in, 1 out]
                            n259 = local read "最终位移上限"() -> (w350:dbl)
                            n260 = local read "最终位移下限"() -> (w349:dbl)
                            n261 = local read "判定结果2"() -> (w343:string)
                            n262 = local read "判定结果3"() -> (w351:string)
                            n263 = Decimal String To Number(string=w336, default (0L)=i64 0 ("默认(0 I32)")) -> (number=w337:i64)  [unwired: 1 in, 1 out]
                            n264 = Decimal String To Number(string=w339, default (0L)=i64 0 ("默认(0 I32)")) -> (number=w338:i64)  [unwired: 1 in, 1 out]
                            n265 = Decimal String To Number(string=w344, default (0L)=i64 0 ("默认(0 I32)")) -> (number=w345:i64)  [unwired: 1 in, 1 out]
                            n266 = Decimal String To Number(string=w347, default (0L)=i64 0 ("默认(0 I32)")) -> (number=w346:i64)  [unwired: 1 in, 1 out]
                            n267 = case shown="2" w316 {
                              tunnel: ["" ("元素") "OK" "NG"] -> w315
                              frame 0, Default {
                              }
                              frame 1 {
                              }
                              frame 2 {
                              }
                            }
                            n268 = Bundle(w337, w338, "位移区间内最小压力", "位移区间内最小压力(KN)"=w340, "最小压力下限"=w341, "最小压力上限"=w342, "KN", "判定结果2"=w343) -> (w327:T5)  [unwired: 1 in]
                            n269 = Bundle(w345, w346, "拉装最终位移", "拉装最终位移(mm)"=w348, "最终位移下限"=w349, "最终位移上限"=w350, "mm", "判定结果3"=w351) -> (w326:T6)  [unwired: 1 in]
                            n270 = local read "位移区间内最大压力(KN)"() -> (w355:dbl)
                            n271 = local read "deviceid"() -> (w325:string)
                            n272 = local read "deviceid"() -> (w361:string)
                            n273 = local read "codeid"() -> (w322:string)
                            n274 = local read "codeid"() -> (w357:string)
                            n275 = local read "最大压力上限"() -> (w353:dbl)
                            n276 = local read "最大压力下限"() -> (w354:dbl)
                            n277 = local read "判定结果1"() -> (w352:string)
                            n278 = global read "Global1.vi" "联机模式"() -> (w370:enum16{"单机", "追溯"})
                            n279 = Decimal String To Number(string=w325, default (0L)=i64 0 ("默认(0 I32)")) -> (number=w324:i64)  [unwired: 1 in, 1 out]
                            n280 = Decimal String To Number(string=w322, default (0L)=i64 0 ("默认(0 I32)")) -> (number=w323:i64)  [unwired: 1 in, 1 out]
                            n281 = Decimal String To Number(string=w361, default (0L)=i64 0 ("默认(0 I32)")) -> (number=w359:i64)  [unwired: 1 in, 1 out]
                            n282 = Decimal String To Number(string=w357, default (0L)=i64 0 ("默认(0 I32)")) -> (number=w358:i64)  [unwired: 1 in, 1 out]
                            n283 = call "GetSQLstring.vi"("联机模式"=w370) -> ("错误输出"=w368:errorcluster, "连接字符串"=w369:string)  [unwired: 9 in]
                            n284 = Bundle(w324, w323, "CCD卡簧检测", w317, w317, w317, "/", "元素"=w315) -> (w314:T7)  [unwired: 1 in]
                            n285 = Bundle(w359, w358, "位移区间内最大压力", "位移区间内最大压力(KN)"=w355, "最大压力下限"=w354, "最大压力上限"=w353, "KN", "判定结果1"=w352) -> (w363:T8)  [unwired: 1 in]
                            n286 = Build Array(w363, w327, w326, w314) -> (w362:T9)
                            n287 = call-poly <vilib>:"DB Tools Open Connection.vi"("error in (no error)"=w368, "connection information"=w369) -> ("error out"=w371:errorcluster, "connection reference"=w366:T10)  [unwired: 6 in]
                            n288 = for {
                              tunnel: w362 -> [w379] mode=indexing
                              tunnel: w366 -> [w377]
                              shift-right: [w375] -> w364
                              shift-left: w371 -> [w382]
                              w378 = string[] ["DEVICE_ID", "CODE_ID", "TEST_NAME", "TEST_VALUE", "TEST_VALUE_MIN", "TEST_VALUE_MAX", "TEST_VALUE_UNIT", "TEST_VALUE_RESULT"] ("columns")
                              w380 = "Test" ("table")
                              n289 = call <vilib>:"DB Tools Insert Data.vi"("data"=w379, "error in (no error)"=w382, "columns"=w378, "table"=w380, "connection reference"=w377) -> ("error out"=w381:errorcluster, "connection reference out"=w376:T10)  [unwired: 5 in]
                              n290 = case shown="错误" w381 {
                                selector: w381 -> [w383 w408]
                                tunnel: w378 -> [_ w405]
                                tunnel: w376 -> [w384 w391]
                                tunnel: w380 -> [_ w409]
                                tunnel: w379 -> [_ w400]
                                tunnel: [w384 w390] -> _
                                tunnel: [w383 w389] -> w375
                                frame No Error {
                                }
                                frame Error {
                                n291 = Delete From Array(array=w405, length=1 ("长度"), index=2 ("索引")) -> (array with subset deleted=w406:string[])  [unwired: 1 out]
                                n292 = call <vilib>:"Clear Errors.vi"("error in (no error)"=w408) -> ("error out"=w407:errorcluster)  [unwired: 5 in, 1 out]
                                n293 = Unbundle(w400) -> (w399:i64, w385:i64, w392:string, "拉装最终位移(mm)"=w398:dbl, "最终位移下限"=w397:dbl, "最终位移上限"=w396:dbl, w395:string, "元素"=w394:string)
                                n294 = Bundle(w399, w385, "拉装最终位移(mm)"=w398, "最终位移下限"=w397, "最终位移上限"=w396, w395, "元素"=w394) -> (w393:T11)  [unwired: 1 in]
                                n295 = Number To Decimal String(number=w385) -> (decimal integer string=w386:string)  [unwired: 1 in]
                                n296 = Concatenate Strings("WHERE TEST_NAME ='" ("condition"), w392, "'", "AND CODE_ID =" ("condition"), w386) -> (w402:string)
                                n297 = call <vilib>:"DB Tools Update Data.vi"("condition"=w402, "data"=w393, "error in (no error)"=w407, "columns"=w406, "table"=w409, "connection reference"=w391) -> ("error out"=w389:errorcluster, "connection reference out"=w390:T10)  [unwired: 4 in]
                                }
                              }
                            }
                            n298 = call <vilib>:"Simple Error Handler.vi"("error in (no error)"=w364) -> ()  [unwired: 4 in, 5 out]
                          }
                          frame #1 {
                            n299 = shared-variable "我的电脑\\160上转向轴拉装.lvlib\\备用_1"(u16 103 ("备用1")) -> ()  [unwired: 1 in, 1 out]
                          }
                        }
                      }
                    }
                  }
                  frame 103 {
                    n300 = global read "Global1.vi" "联机模式"() -> (w411:enum16{"单机", "追溯"})
                    n301 = case shown="\"追溯\"" w411 {
                      frame "单机", Default {
                        n302 = shared-variable "我的电脑\\160上转向轴拉装.lvlib\\备用_1"(u16 0 ("备用1")) -> ()  [unwired: 1 in, 1 out]
                        n303 = shared-variable "我的电脑\\160上转向轴拉装.lvlib\\备用_3"(u16 0 ("备用1")) -> ()  [unwired: 1 in, 1 out]
                      }
                      frame "追溯" {
                        n304 = stacked-sequence {
                          frame #0 {
                            n305 = shared-variable "我的电脑\\160上转向轴拉装.lvlib\\备用_5"() -> (w418:u16)  [unwired: 1 in, 1 out]
                            n306 = Get Date/Time String(date format (0)=enum16{"short", "long", "abbreviated"}."short" ("日期格式(0)"), want seconds? (F)=FALSE ("需要秒？(F)")) -> (date string=w426:string, time string=w425:string)  [unwired: 1 in]
                            n307 = local read "USER_ID"() -> (w415:string)
                            n308 = case shown="1" w418 {
                              tunnel: ["" "OK" "NG"] -> w417
                              frame 0, Default {
                              }
                              frame 1 {
                              }
                              frame 2 {
                              }
                            }
                            n309 = Concatenate Strings(w426, " " ("字符串"), w425) -> (w422:string)
                            n310 = local read "deviceid"() -> (w434:string)
                            n311 = local read "codeid"() -> (w431:string)
                            n312 = global read "Global1.vi" "联机模式"() -> (w441:enum16{"单机", "追溯"})
                            n313 = Search and Replace String(replace all?=TRUE ("替换全部？(F)"), input string=w422, search string="/" ("替换字符串(\"\")"), replace string="-" ("替换字符串(\"\")")) -> (result string=w423:string)  [unwired: 4 in, 3 out]
                            n314 = Decimal String To Number(string=w415, default (0L)=i64 0 ("默认(0 I32)")) -> (number=w414:i64)  [unwired: 1 in, 1 out]
                            n315 = Decimal String To Number(string=w434, default (0L)=i64 0 ("默认(0 I32)")) -> (number=w432:i64)  [unwired: 1 in, 1 out]
                            n316 = Decimal String To Number(string=w431, default (0L)=i64 0 ("默认(0 I32)")) -> (number=w429:i64)  [unwired: 1 in, 1 out]
                            n317 = Bundle(w432, w414, w429, w417, "result string"=w423) -> (w436:T12)  [unwired: 1 in]
                            n318 = call "GetSQLstring.vi"("联机模式"=w441) -> ("错误输出"=w439:errorcluster, "连接字符串"=w440:string)  [unwired: 9 in]
                            n319 = Build Array(w436) -> (w435:T13)
                            n320 = call-poly <vilib>:"DB Tools Open Connection.vi"("error in (no error)"=w439, "connection information"=w440) -> ("error out"=w442:errorcluster, "connection reference"=w438:T10)  [unwired: 6 in]
                            n321 = for {
                              tunnel: w435 -> [w450] mode=indexing
                              tunnel: w438 -> [w448]
                              shift-right: [w446] -> w437
                              shift-left: w442 -> [w453]
                              w449 = string[] ["DEVICE_ID", "USER_ID", "CODE_ID", "RESULT_VALUE", "RESULT_TIME"] ("columns")
                              w451 = "Result" ("table")
                              n322 = call <vilib>:"DB Tools Insert Data.vi"("data"=w450, "error in (no error)"=w453, "columns"=w449, "table"=w451, "connection reference"=w448) -> ("error out"=w452:errorcluster, "connection reference out"=w447:T10)  [unwired: 5 in]
                              n323 = case shown="错误" w452 {
                                selector: w452 -> [w454 w475]
                                tunnel: w449 -> [_ w472]
                                tunnel: w447 -> [w455 w464]
                                tunnel: w451 -> [_ w476]
                                tunnel: w450 -> [_ w468]
                                tunnel: [w455 w463] -> _
                                tunnel: [w454 w462] -> w446
                                frame No Error {
                                }
                                frame Error {
                                n324 = Array Subset(array=w472, index=3 ("长度"), length=2 ("索引")) -> (w473:string[])
                                n325 = Unbundle(w468) -> (w457:i64, w460:i64, w467:string, "result string"=w466:string)  [unwired: 1 out]
                                n326 = Bundle(w467, "result string"=w466) -> (w465:cluster{string, "result string":string})  [unwired: 1 in]
                                n327 = Number To Decimal String(number=w460) -> (decimal integer string=w461:string)  [unwired: 1 in]
                                n328 = Number To Decimal String(number=w457) -> (decimal integer string=w456:string)  [unwired: 1 in]
                                n329 = call <vilib>:"Clear Errors.vi"("error in (no error)"=w475) -> ("error out"=w474:errorcluster)  [unwired: 5 in, 1 out]
                                n330 = Concatenate Strings("WHERE CODE_ID =" ("condition"), w461, "AND DEVICE_ID =", w456) -> (w469:string)
                                n331 = call <vilib>:"DB Tools Update Data.vi"("condition"=w469, "data"=w465, "error in (no error)"=w474, "columns"=w473, "table"=w476, "connection reference"=w464) -> ("error out"=w462:errorcluster, "connection reference out"=w463:T10)  [unwired: 4 in]
                                }
                              }
                            }
                            n332 = call <vilib>:"Simple Error Handler.vi"("error in (no error)"=w437) -> ()  [unwired: 4 in, 5 out]
                          }
                          frame #1 {
                            n333 = shared-variable "我的电脑\\160上转向轴拉装.lvlib\\备用_1"(u16 0 ("备用1")) -> ()  [unwired: 1 in, 1 out]
                            n334 = shared-variable "我的电脑\\160上转向轴拉装.lvlib\\备用_3"(u16 0 ("备用1")) -> ()  [unwired: 1 in, 1 out]
                          }
                        }
                      }
                    }
                  }
                  frame 1000 {
                    n335 = stacked-sequence {
                      frame #0 {
                        n336 = shared-variable "我的电脑\\Global.lvlib\\工位追溯码"("" ("传感器码")) -> ()  [unwired: 1 in, 1 out]
                        n337 = Wait (ms)(milliseconds to wait=u32 300 ("等待时间（毫秒）")) -> ()  [unwired: 1 out]
                        n338 = local write "上序状态显示"("" ("上序状态显示")) -> ()
                        n339 = property on="上序状态" class="Bool (严格)"("Colors [4]"=cluster{u32, u32}[] [{11776947, 11776947}, {11776947, 11776947}, {11776947, 11776947}, {11776947, 11776947}] ("颜色[4]")) -> ()  [unwired: 2 in, 2 out]
                      }
                      frame #1 {
                        w485 = "请扫码！" ("通知内容")
                        n340 = call "输入框.vi"("提示信息"=w485) -> ("条形码输出"=w484:string)
                        "产品条码" <- w484
                        n341 = call "浮动通知.vi"("通知内容"=w485) -> ()  [unwired: 11 in]
                        n342 = shared-variable "我的电脑\\160上转向轴拉装.lvlib\\备用_1"(u16 1001 ("备用1")) -> ()  [unwired: 1 in, 1 out]
                        n343 = shared-variable "我的电脑\\Global.lvlib\\工位追溯码"(w484) -> ()  [unwired: 1 in, 1 out]
                      }
                    }
                  }
                  frame 1001 {
                    n344 = shared-variable "我的电脑\\Global.lvlib\\工位追溯码"() -> (w486:string)  [unwired: 1 in, 1 out]
                    n345 = String Length(string=w486) -> (length=w488:i32)
                    n346 = Greater?(x=w488, y=4) -> (0:w489:bool)
                    n347 = case shown="真" w489 {
                      frame False {
                      }
                      frame True {
                        n348 = shared-variable "我的电脑\\160上转向轴拉装.lvlib\\备用_1"(u16 1100 ("备用1")) -> ()  [unwired: 1 in, 1 out]
                      }
                    }
                  }
                  frame 1100 {
                    n349 = global read "Global1.vi" "联机模式"() -> (w491:enum16{"单机", "追溯"})
                    n350 = case shown="\"追溯\"" w491 {
                      frame "单机", Default {
                        n351 = shared-variable "我的电脑\\160上转向轴拉装.lvlib\\备用_1"(u16 1002 ("备用1")) -> ()  [unwired: 1 in, 1 out]
                      }
                      frame "追溯" {
                        n352 = stacked-sequence {
                          frame #0 {
                            n353 = shared-variable "我的电脑\\Global.lvlib\\工位追溯码"() -> (w499:string)  [unwired: 1 in, 1 out]
                            n354 = local read "productid"() -> (w497:string)
                            n355 = global read "Global1.vi" "联机模式"() -> (w514:enum16{"单机", "追溯"})
                            n356 = call "GetSQLstring.vi"("联机模式"=w514) -> ("错误输出"=w512:errorcluster, "连接字符串"=w513:string)  [unwired: 9 in]
                            n357 = Concatenate Strings("SELECT CODE_ID  FROM CODE  WHERE CODE_MAIN ='", w499, "'" ("字符串"), " AND PRODUCT_ID='", w497, "'" ("字符串")) -> (w511:string)
                            n358 = call-poly <vilib>:"DB Tools Open Connection.vi"("error in (no error)"=w512, "connection information"=w513) -> ("error out"=w505:errorcluster, "connection reference"=w506:T10)  [unwired: 6 in]
                            n359 = call-poly <vilib>:"DB Tools Execute Query.vi"("error in (no error)"=w505, "SQL query"=w511, "connection reference"=w506) -> ("error out"=w509:errorcluster, "recordset reference"=w510:T14)  [unwired: 5 in]
                            n360 = call-poly <vilib>:"DB Tools Fetch Recordset Data.vi"("error in (no error)"=w509, "recordset reference"=w510) -> ("error out"=w504:errorcluster, "recordset data"=w508:variant[][])  [unwired: 3 in, 1 out]
                            n361 = Variant To Data(error in=w504, type=string[][] [], Variant=w508) -> (data=w503:string[][])  [unwired: 1 out]
                            n362 = Index Array(array=w503, index (row)=0 ("索引 (行)")) -> (element=w501:string[])  [unwired: 1 in]
                            n363 = Index Array(array=w501, index=0 ("索引 (行)")) -> (element=w493:string)
                            n364 = local write "codeid"(w493) -> ()
                            n365 = case shown="\"\"" w493 {
                              frame "假", Default {
                              }
                              frame "" {
                                n366 = shared-variable "我的电脑\\160上转向轴拉装.lvlib\\备用_1"(u16 5000 ("备用1")) -> ()  [unwired: 1 in, 1 out]
                                n367 = local write "上序状态显示"("漏序" ("上序状态显示")) -> ()
                                n368 = property on="上序状态" class="Bool (严格)"("Colors [4]"=cluster{u32, u32}[] [{16767232, 16767232}, {16767232, 16767232}, {16767232, 16767232}, {16767232, 16767232}] ("颜色[4]")) -> ()  [unwired: 2 in, 2 out]
                              }
                            }
                          }
                          frame #1 {
                            n369 = local read "Fdeviceid"() -> (w521:string)
                            n370 = local read "codeid"() -> (w522:string)
                            n371 = global read "Global1.vi" "联机模式"() -> (w538:enum16{"单机", "追溯"})
                            n372 = call "GetSQLstring.vi"("联机模式"=w538) -> ("错误输出"=w536:errorcluster, "连接字符串"=w537:string)  [unwired: 9 in]
                            n373 = Concatenate Strings("SELECT RESULT_VALUE FROM RESULT  WHERE DEVICE_ID =\n" ("table"), w521, " AND CODE_ID ='" ("字符串"), w522, "'" ("字符串")) -> (w535:string)
                            n374 = call-poly <vilib>:"DB Tools Open Connection.vi"("error in (no error)"=w536, "connection information"=w537) -> ("error out"=w529:errorcluster, "connection reference"=w530:T10)  [unwired: 6 in]
                            n375 = call-poly <vilib>:"DB Tools Execute Query.vi"("error in (no error)"=w529, "SQL query"=w535, "connection reference"=w530) -> ("error out"=w533:errorcluster, "recordset reference"=w534:T14)  [unwired: 5 in]
                            n376 = call-poly <vilib>:"DB Tools Fetch Recordset Data.vi"("error in (no error)"=w533, "recordset reference"=w534) -> ("error out"=w528:errorcluster, "recordset data"=w532:variant[][])  [unwired: 3 in, 1 out]
                            n377 = Variant To Data(error in=w528, type=string[][] [], Variant=w532) -> (data=w524:string[][])  [unwired: 1 out]
                            n378 = Index Array(array=w524, index (row)=0 ("索引 (行)")) -> (element=w526:string[])  [unwired: 1 in]
                            n379 = Index Array(array=w526, index=0 ("索引 (行)")) -> (element=w523:string)
                            n380 = case shown="\"NG\"" w523 {
                              frame "假", Default {
                              }
                              frame "OK" {
                                n381 = local write "上序状态显示"("合格" ("上序状态显示")) -> ()
                                n382 = shared-variable "我的电脑\\160上转向轴拉装.lvlib\\备用_1"(u16 1002 ("备用1")) -> ()  [unwired: 1 in, 1 out]
                                n383 = property on="上序状态" class="Bool (严格)"("Colors [4]"=cluster{u32, u32}[] [{6618880, 6618880}, {6618880, 6618880}, {6618880, 6618880}, {6618880, 6618880}] ("颜色[4]")) -> ()  [unwired: 2 in, 2 out]
                              }
                              frame "NG" {
                                n384 = local write "上序状态显示"("不合格" ("上序状态显示")) -> ()
                                n385 = shared-variable "我的电脑\\160上转向轴拉装.lvlib\\备用_1"(u16 5000 ("备用1")) -> ()  [unwired: 1 in, 1 out]
                                n386 = property on="上序状态" class="Bool (严格)"("Colors [4]"=cluster{u32, u32}[] [{16711680, 16711680}, {16711680, 16711680}, {16711680, 16711680}, {16711680, 16711680}] ("颜色[4]")) -> ()  [unwired: 2 in, 2 out]
                              }
                            }
                          }
                        }
                      }
                    }
                  }
                }
              }
            }
          }
          event "删除": Value Change {
            n387 = event-data() -> ("NewVal"=w545:bool)  [unwired: 1 in, 5 out]
            n388 = case shown="真" w545 {
              tunnel: w546 -> [_ w548]
              frame False {
              }
              frame True {
                n389 = Concatenate Strings("确认删除“", "请选择要删除的产品", "”吗？") -> (w550:string)
                n390 = Two Button Dialog(message=w550) -> (T button?=w549:bool)  [unwired: 2 in]
                n391 = case shown="真" w549 {
                  tunnel: w548 -> [_ w554]
                  tunnel: "请选择要删除的产品" -> [_ w553]
                  frame False {
                  }
                  frame True {
                    n392 = call <vilib>:"Open Config Data.vi"("configuration file path"=w554) -> ("error out"=w556:errorcluster, "refnum"=w559:T4)  [unwired: 8 in, 1 out]
                    n393 = call <vilib>:"Remove Section.vi"("section"=w553, "error in (no error)"=w556, "refnum"=w559) -> ("error out"=w558:errorcluster, "section exists?"=w555:bool, "refnum out"=w557:T4)  [unwired: 6 in]
                    n394 = call <vilib>:"Close Config Data.vi"("error in (no error)"=w558, "refnum"=w557) -> ()  [unwired: 8 in, 2 out]
                    n395 = case shown="真" w555 {
                      frame False {
                        n396 = One Button Dialog(message="删除失败！\n请确认产品存在！" ("消息")) -> ()  [unwired: 1 in, 1 out]
                      }
                      frame True {
                        n397 = One Button Dialog(message="删除成功！" ("消息")) -> ()  [unwired: 1 in, 1 out]
                      }
                    }
                  }
                }
              }
            }
          }
          event "确定": Value Change {
            n398 = event-data() -> ("NewVal"=w562:bool)  [unwired: 1 in, 5 out]
            n399 = case shown="真" w562 {
              frame False {
              }
              frame True {
                n400 = stacked-sequence {
                  seq-local: [w566 _ _ _ _ _] -> [_ _ _ _ _ _]
                  frame #0 {
                    n401 = global read "Global1.vi" "联机模式"() -> (w563:enum16{"单机", "追溯"})
                    n402 = case shown="\"追溯\"" w563 {
                      frame "单机", Default {
                      }
                      frame "追溯" {
                        n403 = local read "产品型号"() -> (w573:string)
                        n404 = call "Get_Device_ID.vi"() -> ("Device_ID"=→"deviceid":string)  [unwired: 10 in, 1 out]
                        n405 = call "GET_PRODUCT_ID.vi"("PRODFUCT_NAME"=w573) -> ("PRODUCT_ID"=w572:string)  [unwired: 10 in]
                        "productid" <- w572
                        n406 = call "查询前序设备.vi"("PRODUCT_ID"=w572) -> ("前序工位"=w571:string[])  [unwired: 10 in]
                        n407 = Index Array(array=w571, index=0 ("索引")) -> (element=→"Fdeviceid":string)
                      }
                    }
                    n408 = local read "产品型号"() -> (w565:string)
                    "产品型号" <- w565
                    n409 = shared-variable "我的电脑\\Global.lvlib\\产品型号"(w565) -> ()  [unwired: 1 in, 1 out]
                    n410 = String Subset(string=w565, offset (0)=u16 2 ("偏移量(0)"), length (rest)=u16 4 ("长度（剩余）")) -> (substring=w566:string)
                    n411 = property on="选项卡控件 2" class="TabCtl (严格)"("Value"=enum32{"上转向轴拉装曲线", "参数查看"}."上转向轴拉装曲线" ("选项卡控件 2")) -> ()  [unwired: 2 in, 2 out]
                    n412 = Decimal String To Number(string=w566) -> ()  [unwired: 2 in, 2 out]
                  }
                  frame #1 {
                    n413 = local read "用户名"() -> (w575:string)
                    n414 = global read "Global1.vi" "联机模式"() -> (w582:enum16{"单机", "追溯"})
                    n415 = call "GetSQLstring.vi"("联机模式"=w582) -> ("错误输出"=w584:errorcluster, "连接字符串"=w583:string)  [unwired: 9 in]
                    n416 = call-poly <vilib>:"DB Tools Open Connection.vi"("error in (no error)"=w584, "connection information"=w583) -> ("error out"=w590:errorcluster, "connection reference"=w589:T10)  [unwired: 6 in]
                    n417 = Concatenate Strings("SELECT USER_ID FROM [User]  WHERE USER_NAME ='", w575, "'" ("字符串")) -> (w585:string)
                    n418 = call-poly <vilib>:"DB Tools Execute Query.vi"("error in (no error)"=w590, "SQL query"=w585, "connection reference"=w589) -> ("error out"=w587:errorcluster, "recordset reference"=w586:T14)  [unwired: 5 in]
                    n419 = call-poly <vilib>:"DB Tools Fetch Recordset Data.vi"("error in (no error)"=w587, "recordset reference"=w586) -> ("error out"=w591:errorcluster, "recordset data"=w588:variant[][])  [unwired: 3 in, 1 out]
                    n420 = Variant To Data(error in=w591, type=string[][] [], Variant=w588) -> (data=w592:string[][])  [unwired: 1 out]
                    n421 = Index Array(array=w592, index (row)=0 ("索引 (行)")) -> (element=w593:string[])  [unwired: 1 in]
                    n422 = Index Array(array=w593, index=0 ("索引 (行)")) -> (element=→"USER_ID":string)
                  }
                  frame #2 {
                    n423 = local read "坐标轴参数"() -> (w598:string[][])
                    n424 = Index Array(array=w598, index (row) #1=0 ("索引 (行)"), index (row) #2=1 ("索引 (行)"), index (row) #3=2 ("索引 (行)"), index (row) #4=3 ("索引 (行)")) -> (element #1=w610:string[], element #2=w605:string[], element #3=w604:string[], element #4=w603:string[])  [unwired: 4 in]
                    n425 = Index Array(array=w610, index=1 ("索引")) -> (element=w602:string)
                    n426 = Index Array(array=w605, index=1 ("索引")) -> (element=w601:string)
                    n427 = Index Array(array=w604, index=1 ("索引")) -> (element=w600:string)
                    n428 = Index Array(array=w603, index=1 ("索引")) -> (element=w599:string)
                    n429 = Fract/Exp String To Number(string=w599) -> (number=w594:dbl)  [unwired: 3 in, 1 out]
                    n430 = Fract/Exp String To Number(string=w600) -> (number=w595:dbl)  [unwired: 3 in, 1 out]
                    n431 = Fract/Exp String To Number(string=w601) -> (number=w596:dbl)  [unwired: 3 in, 1 out]
                    n432 = Fract/Exp String To Number(string=w602) -> (number=w597:dbl)  [unwired: 3 in, 1 out]
                    n433 = property on="拉力位移曲线" class="XYGraph (严格)"("XScale.Minimum"=w597) -> ()  [unwired: 2 in, 2 out]
                    n434 = property on="拉力位移曲线" class="XYGraph (严格)"("XScale.Maximum"=w596) -> ()  [unwired: 2 in, 2 out]
                    n435 = property on="拉力位移曲线" class="XYGraph (严格)"("YScale.Minimum"=w595) -> ()  [unwired: 2 in, 2 out]
                    n436 = property on="拉力位移曲线" class="XYGraph (严格)"("YScale.Maximum"=w594) -> ()  [unwired: 2 in, 2 out]
                  }
                  frame #3 {
                    n437 = local read "判定框参数"() -> (w624:string[][])
                    n438 = Index Array(array=w624, index (row) #1=0 ("索引 (行)"), index (row) #2=1 ("索引 (行)"), index (row) #3=2 ("索引 (行)"), index (row) #4=3 ("索引 (行)")) -> (element #1=w632:string[], element #2=w627:string[], element #3=w626:string[], element #4=w625:string[])  [unwired: 4 in]
                    n439 = Index Array(array=w632, index=1 ("索引")) -> (element=w619:string)
                    n440 = Index Array(array=w627, index=1 ("索引")) -> (element=w618:string)
                    n441 = Index Array(array=w626, index=1 ("索引")) -> (element=w617:string)
                    n442 = Index Array(array=w625, index=1 ("索引")) -> (element=w616:string)
                    n443 = local read "拉力位移曲线"() -> (w637:cluster{dbl[], dbl[]}[])
                    n444 = Fract/Exp String To Number(string=w616) -> (number=w621:dbl)  [unwired: 3 in, 1 out]
                    n445 = Fract/Exp String To Number(string=w617) -> (number=w620:dbl)  [unwired: 3 in, 1 out]
                    n446 = Fract/Exp String To Number(string=w618) -> (number=w622:dbl)  [unwired: 3 in, 1 out]
                    n447 = Fract/Exp String To Number(string=w619) -> (number=w623:dbl)  [unwired: 3 in, 1 out]
                    n448 = for {
                      tunnel: [w644] -> w615 mode=indexing
                      tunnel: w637 -> [w643] mode=indexing
                      tunnel: w623 -> [w641]
                      tunnel: w622 -> [w640]
                      tunnel: w621 -> [w639]
                      tunnel: w620 -> [w638]
                      i -> [w642]
                      n449 = case shown="0" w642 {
                        tunnel: [w645 w650] -> w644
                        tunnel: w643 -> [w645 _]
                        tunnel: w641 -> [_ w649]
                        tunnel: w640 -> [_ w648]
                        tunnel: w639 -> [_ w647]
                        tunnel: w638 -> [_ w646]
                        frame Default {
                        }
                        frame 0 {
                          n450 = Build Array(w649, w649, w648, w648, w649) -> (w651:dbl[])
                          n451 = Build Array(w646, w647, w647, w646, w646) -> (w652:dbl[])
                          n452 = Bundle(w651, w652) -> (w650:cluster{dbl[], dbl[]})  [unwired: 1 in]
                        }
                      }
                    }
                    n453 = local write "拉力位移曲线"(w615) -> ()
                  }
                  frame #4 {
                    n454 = local read "结果判定参数"() -> (w658:string[][])
                    n455 = local read "判定框参数"() -> (w655:string[][])
                    n456 = Index Array(array=w655, index (row) #1=2 ("索引 (行)"), index (row) #2=3 ("索引 (行)")) -> (element #1=w672:string[], element #2=w670:string[])  [unwired: 2 in]
                    n457 = Index Array(array=w658, index (row) #1=0 ("索引 (行)"), index (row) #2=0 ("索引 (行)")) -> (element #1=w664:string[], element #2=w662:string[])  [unwired: 2 in]
                    n458 = Index Array(array=w672, index=1 ("索引")) -> (element=w668:string)
                    n459 = Index Array(array=w670, index=1 ("索引")) -> (element=w667:string)
                    n460 = Index Array(array=w664, index=1 ("索引")) -> (element=w660:string)
                    n461 = Index Array(array=w662, index=2 ("索引")) -> (element=w659:string)
                    n462 = Fract/Exp String To Number(string=w668) -> (number=w653:dbl)  [unwired: 3 in, 1 out]
                    n463 = Fract/Exp String To Number(string=w667) -> (number=w654:dbl)  [unwired: 3 in, 1 out]
                    n464 = Fract/Exp String To Number(string=w660) -> (number=w656:dbl)  [unwired: 3 in, 1 out]
                    n465 = Fract/Exp String To Number(string=w659) -> (number=w657:dbl)  [unwired: 3 in, 1 out]
                    n466 = local write "最大压力上限"(w654) -> ()
                    n467 = local write "最小压力上限"(w654) -> ()
                    n468 = local write "最小压力下限"(w653) -> ()
                    n469 = local write "最大压力下限"(w653) -> ()
                    n470 = local write "最终位移下限"(w656) -> ()
                    n471 = local write "最终位移上限"(w657) -> ()
                  }
                  frame #5 {
                    w675 = "参数装载成功！" ("消息")
                    n472 = One Button Dialog(message=w675) -> ()  [unwired: 1 in, 1 out]
                    n473 = call "浮动通知.vi"("通知内容"=w675) -> ()  [unwired: 11 in]
                  }
                }
              }
            }
          }
          event "添加": Value Change {
            n474 = event-data() -> ("NewVal"=w678:bool)  [unwired: 1 in, 5 out]
            n475 = local read "请输入添加的产品名称"() -> (w676:string)
            n476 = call <vilib>:"Trim Whitespace.vi"("string"=w676) -> ("trimmed string"=w680:string)  [unwired: 1 in]
            n477 = White Space?(1:w680) -> (0:w681:bool)
            n478 = case shown="假" w681 {
              tunnel: w677 -> [w684 _]
              tunnel: w678 -> [w683 _]
              tunnel: w679 -> [w682 _]
              frame False {
                n479 = case shown="真" w683 {
                  tunnel: w684 -> [_ w686]
                  tunnel: w682 -> [_ w685]
                  frame False {
                  }
                  frame True {
                    n480 = for {
                      tunnel: w686 -> [w689] mode=indexing
                      tunnel: w685 -> [w688]
                      n481 = call "Read_Write ParaINI File.vi"("Mode"=enum16{"Read", "Write"}."Write", "Section"="请输入添加的产品名称", "Filepath"=w688, "Ctl Refnum"=w689) -> ()  [unwired: 7 in, 1 out]
                    }
                  }
                }
              }
              frame True {
                w691 = 64 items=["None"=0, "Hand, Error, Stop"=16, "Question"=32, "Exclamation, Warning"=48, "Asterisk, Information"=64] ("icon")
                w692 = 0 items=["OK", "OKCancel", "AbortRetryIgnore", "YesNoCancel", "YesNo", "RetryCancel"] ("buttons")
                n482 = call "信息框（标题、文本、图标）.vi"("icon"=w691, "buttons"=w692, "caption"="添加失败", "text"="请输入产品名称!") -> ()  [unwired: 6 in, 2 out]
              }
            }
          }
          event "产品型号": Value Change {
            n483 = event-data() -> ()  [unwired: 1 in, 6 out]
            n484 = stacked-sequence {
              tunnel: w695 -> [_ w698]
              tunnel: w696 -> [_ w697]
              frame #0 {
              }
              frame #1 {
                n485 = for {
                  tunnel: w698 -> [w701] mode=indexing
                  tunnel: w697 -> [w700]
                  n486 = local read "产品型号"() -> (w699:string)
                  n487 = call "Read_Write ParaINI File.vi"("Mode"=enum16{"Read", "Write"}."Read", "Section"=w699, "Filepath"=w700, "Ctl Refnum"=w701) -> ()  [unwired: 7 in, 1 out]
                }
              }
            }
          }
          event "退出": Value Change {
            n488 = event-data() -> ()  [unwired: 1 in, 6 out]
            n489 = control-ref of="本VI"() -> (w705:refnum<vi>)
            n490 = invoke class="VI" method="FP.Close"(reference=w705) -> (reference out=w703:refnum<vi>, error out=w704:errorcluster)  [unwired: 2 in, 1 out]
            n491 = Close Reference(reference=w703, error in (no error)=w704) -> ()  [unwired: 1 out]
          }
          event "更新": Value Change {
            n492 = event-data() -> ("NewVal"=w708:bool)  [unwired: 1 in, 5 out]
            n493 = case shown="真" w708 {
              tunnel: w707 -> [_ w711]
              tunnel: w706 -> [_ w710]
              frame False {
              }
              frame True {
                n494 = for {
                  tunnel: w711 -> [w717]
                  tunnel: w710 -> [w716] mode=indexing
                  tunnel: [w715] -> w709
                  n495 = local read "产品型号"() -> (w714:string)
                  n496 = call "Read_Write ParaINI File.vi"("Mode"=enum16{"Read", "Write"}."Write", "Section"=w714, "Filepath"=w717, "Ctl Refnum"=w716) -> ("error out"=w715:errorcluster)  [unwired: 7 in]
                }
                n497 = case shown="无错误" w709 {
                  frame No Error {
                    n498 = call "浮动通知.vi"("通知内容"="更新成功！") -> ()  [unwired: 11 in]
                  }
                  frame Error {
                    n499 = call "浮动通知.vi"("通知内容"="更新失败！") -> ()  [unwired: 11 in]
                  }
                }
              }
            }
          }
          event "请输入添加的产品名称": Value Change {
            n500 = event-data() -> ("NewVal"=w720:string)  [unwired: 1 in, 5 out]
            n501 = control-ref of="产品型号"() -> (w719:refnum<vi>)
            n502 = property on="属性节点" class="CmbBox"(reference=w719) -> ("Strings[]"=w721:string[])  [unwired: 1 in, 2 out]
            n503 = for {
              tunnel: w720 -> [w722]
              tunnel: w721 -> [w723] mode=indexing
              n504 = Equal?(x=w722, y=w723) -> (x = y?=w724:bool)
              n505 = case shown="真" w724 {
                tunnel: w722 -> [_ w725]
                frame False {
                }
                frame True {
                  n506 = stacked-sequence {
                    tunnel: w725 -> [w731 _]
                    frame #0 {
                      w726 = 64 items=["None"=0, "Hand, Error, Stop"=16, "Question"=32, "Exclamation, Warning"=48, "Asterisk, Information"=64] ("icon")
                      w727 = 0 items=["OK", "OKCancel", "AbortRetryIgnore", "YesNoCancel", "YesNo", "RetryCancel"] ("buttons")
                      n507 = Concatenate Strings("已经存在产品”" ("text"), w731, "“\n请勿重复添加！" ("字符串")) -> (w729:string)
                      n508 = call "信息框（标题、文本、图标）.vi"("icon"=w726, "buttons"=w727, "caption"="产品重复", "text"=w729) -> ()  [unwired: 6 in, 2 out]
                    }
                    frame #1 {
                      n509 = local write "请输入添加的产品名称"("" ("请输入添加的产品名称")) -> ()
                    }
                  }
                }
              }
            }
          }
          event Panel Close? {
            n510 = event-data() -> ()  [unwired: 1 in, 4 out]
            n511 = global write "Global.vi" "程序关闭"(TRUE ("程序关闭")) -> ()
            n512 = vi-ref "client.vi"() -> (w734:refnum<vi>)
            n513 = control-ref of="本VI"() -> (w739:refnum<vi>)
            n514 = invoke class="VI" method="FP.Close"(reference=w734) -> (reference out=w735:refnum<vi>, error out=w736:errorcluster)  [unwired: 2 in, 1 out]
            n515 = invoke class="VI" method="FP.Close"(reference=w739) -> (reference out=w737:refnum<vi>, error out=w738:errorcluster)  [unwired: 2 in, 1 out]
            n516 = Close Reference(reference=w735, error in (no error)=w736) -> ()  [unwired: 1 out]
            n517 = Close Reference(reference=w737, error in (no error)=w738) -> ()  [unwired: 1 out]
            n518 = event-data("Discard?"=TRUE ("放弃？")) -> ()  [unwired: 1 in, 1 out]
          }
          event "进入用户管理": Value Change {
            n519 = event-data() -> ()  [unwired: 1 in, 6 out]
            n520 = vi-ref "User_manager.vi"() -> (w743:refnum<vi>)
            n521 = call "CallVI.vi"("VI引用"=w743, "状态"=T1."Maximized") -> ()  [unwired: 11 in, 3 out]
          }
          event "设备故障": Value Change {
            n522 = event-data() -> ()  [unwired: 1 in, 6 out]
            n523 = call "状态改变.vi"("设备状态"=enum16{"设备离线", "设备正常", "设备缺料", "设备故障", "质量报警"}."设备故障") -> ()  [unwired: 11 in]
          }
          event "设备缺料": Value Change {
            n524 = event-data() -> ()  [unwired: 1 in, 6 out]
            n525 = call "状态改变.vi"("设备状态"=enum16{"设备离线", "设备正常", "设备缺料", "设备故障", "质量报警"}."设备缺料") -> ()  [unwired: 11 in]
          }
          event "质量报警": Value Change {
            n526 = event-data() -> ()  [unwired: 1 in, 6 out]
            n527 = call "状态改变.vi"("设备状态"=enum16{"设备离线", "设备正常", "设备缺料", "设备故障", "质量报警"}."质量报警") -> ()  [unwired: 11 in]
          }
        }
        n528 = global read "Global.vi" "程序关闭"() -> (w75:bool)
      }
    }
  }
